vi "ActorVaild.vi"(8 "error in (no error)":errorcluster, 10 "name":string, 11 "ActorMap in":refnum<class "ActorMap.lvclass">) -> (0 "error out":errorcluster, 2 "vaild?":bool, 3 "ActorMap out":refnum<class "ActorMap.lvclass">)   [LabVIEW 2020, in "ActorMap.lvclass"]
uses:
  ActorMap.lvclass
  ActorMap.lvclass/ActorMap.ctl
  <vilib>/ActorFramework/Message/Message.lvclass
  <vilib>/ActorFramework/Message Enqueuer/Message Enqueuer.lvclass/Message Enqueuer.ctl
  <vilib>/ActorFramework/Message Priority Queue/Priority Enqueue.vi
  <vilib>/ActorFramework/Message Enqueuer/Message Enqueuer.lvclass
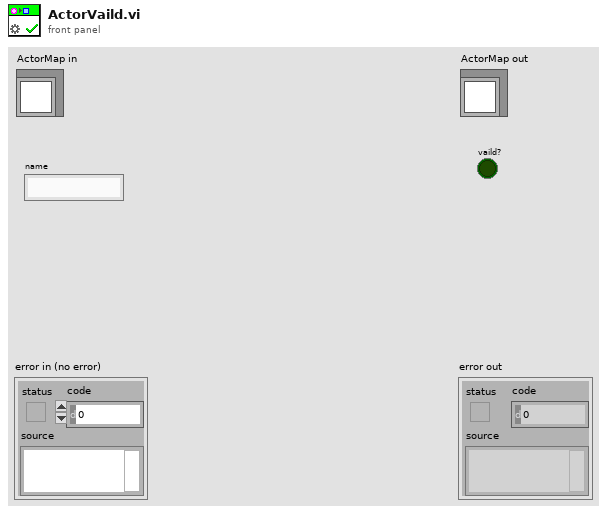
[diagram p1: front panel]
types:
  T1 = map{string, refnum<class "Message Enqueuer.lvclass">}
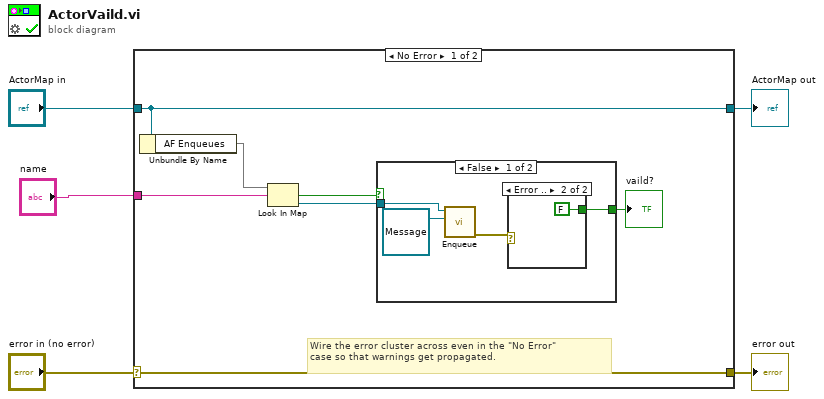
[diagram p0: block diagram]
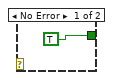
[diagram p2: hidden frame]
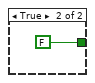
[diagram p3: hidden frame]
diagram:
  n1 = case shown="No Error" "error in (no error)" {
    selector: "error in (no error)" -> [w12 w21]
    tunnel: [w12 w21] -> w4
    tunnel: [w11 w20] -> w2
    tunnel: "ActorMap in" -> [w11 w20]
    tunnel: "name" -> [w9 _]
    frame No Error {
      # "Wire the error cluster across even in the \"No Error\"\ncase so that warnings get propagated."
      n2 = Unbundle By Name(w11) -> ("AF Enqueues"=w10:T1)
      n3 = Look In Map(map=w10, key=w9) -> (key not found?=w7:bool, value=w8:refnum<class "Message Enqueuer.lvclass">)  [unwired: 1 in]
      n4 = case shown="False" w7 {
        tunnel: w8 -> [w16 _]
        tunnel: [w13 FALSE] -> w6
        frame False {
          n5 = call <vilib>:"Enqueue.vi"("Message"=refnum<class "Message.lvclass"> refnum, "Message Enqueuer in"=w16) -> ("error out"=w14:errorcluster)  [unwired: 8 in, 1 out]
          n6 = case shown="Error .." w14 {
            tunnel: [TRUE FALSE] -> w13
            frame No Error {
            }
            frame Error {
            }
          }
        }
        frame True {
        }
      }
      "vaild?" <- w6
    }
    frame Error {
    }
  }
  "error out" <- w4
  "ActorMap out" <- w2
